vi "Lin_SCUBoot.vi"() -> (2 "Data":T1 {"payload" format="%02x"; "identifier" format="%x"})   [LabVIEW 2018]
uses:
  Crl/LIN_DataType.ctl
panel:
  # "ms"
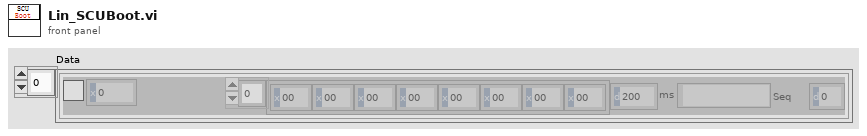
[diagram p1: front panel]
types:
  T1 = typedef "LIN_DataType.ctl" = cluster{"identifier":u32, "payload":u8[], "Send?":bool, "Note":string, "Delays":u32, "Seq":i32}[]
  T2 = cluster{"identifier":u32, "payload":u8[], "Send?":bool, "Note":string, "Delays":u32, "Seq":i32}
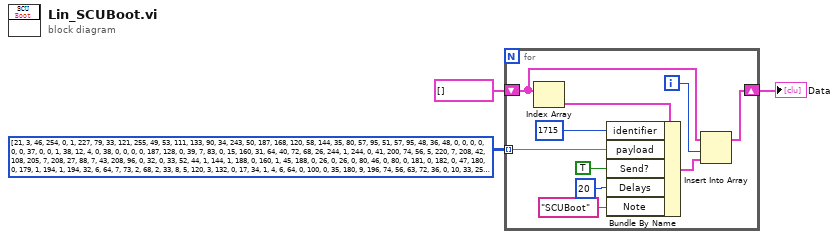
[diagram p0: block diagram]
diagram:
  n1 = for {
    tunnel: u8[][] [[21, 3, 46, 254, 0, 1, 227, 79], [33, 121, 255, 49, 53, 111, 133, 90], [34, 243, 50, 187, 168, 120, 58, 144], [35, 80, 57, 95, 51, 57, 95, 48], [36, 48, 0, 0, 0, 0, 0, 0], [37, 0, 0, 1, 38, 12, 4, 0], [38, 0, 0, 0, 0, 187, 128, 0], [39, 7, 83, 0, 15, 160, 31, 64], [40, 72, 68, 26, 244, 1, 244, 0], [41, 200, 74, 56, 5, 220, 7, 208], [42, 108, 205, 7, 208, 27, 88, 7], [43, 208, 96, 0, 32, 0, 33, 52], [44, 1, 144, 1, 188, 0, 160, 1], [45, 188, 0, 26, 0, 26, 0, 80], [46, 0, 80, 0, 181, 0, 182, 0], [47, 180, 0, 179, 1, 194, 1, 194], [32, 6, 64, 7, 73, 2, 68, 2], [33, 8, 5, 120, 3, 132, 0, 17], [34, 1, 4, 6, 64, 0, 100, 0], [35, 180, 9, 196, 74, 56, 63, 72], [36, 0, 10, 33, 252, 1, 244, 4], [37, 26, 70, 80, 63, 72, 34, 196], [38, 6, 64, 26, 244, 58, 152, 0], [39, 10, 39, 16, 0, 250, 255, 10], [40, 32, 2, 1, 0, 10, 2, 1], [41, 3, 1, 1, 1, 2, 2, 3], [42, 40, 8, 8, 165, 19, 130, 140], [43, 15, 126, 3, 3, 9, 9, 160], [44, 0, 100, 0, 40, 255, 216, 0], [45, 17, 6, 152, 93, 192, 6, 12], [46, 192, 0, 0, 100, 0, 15, 255], [47, 216, 0, 17, 8, 245, 93, 192], [32, 6, 12, 224, 0, 19, 136, 0], [33, 40, 255, 216, 0, 15, 18, 237], [34, 125, 0, 6, 12, 224, 0, 1], [35, 144, 117, 139, 142, 225, 10, 14], [36, 109, 6, 222, 88, 74, 170, 110], [37, 202, 234, 0, 1, 74, 0, 250], [38, 50, 50, 23, 112, 70, 80, 0], [39, 90, 0, 255, 5, 0, 0, 0], [40, 0, 0, 0, 150, 1, 144, 50], [41, 50, 0, 0, 0, 0, 0, 0], [42, 0, 255, 30, 0, 0, 0, 0], [43, 0, 1, 74, 0, 250, 50, 50], [44, 0, 0, 0, 0, 0, 130, 0], [45, 255, 30, 0, 0, 0, 0, 0], [46, 0, 75, 0, 0, 55, 255, 0], [47, 0, 0, 0, 0, 0, 0, 255], [32, 10, 0, 0, 0, 0, 0, 6], [33, 152, 0, 180, 50, 50, 0, 0], [34, 0, 0, 0, 130, 0, 255, 5], [35, 0, 0, 0, 0, 0, 0, 180], [36, 0, 45, 50, 50, 0, 0, 0], [37, 0, 0, 90, 0, 255, 10, 0], [38, 0, 0, 0, 0, 0, 180, 0], [39, 45, 50, 50, 0, 0, 0, 0], [40, 0, 110, 0, 255, 30, 0, 0], [41, 0, 0, 0, 0, 100, 0, 55], [42, 0, 55, 0, 0, 0, 0, 0], [43, 0, 0, 255, 250, 3, 0, 0], [44, 0, 0, 0, 180, 0, 45, 50], [45, 50, 0, 0, 0, 0, 0, 105], [46, 0, 255, 10, 0, 0, 0, 0], [47, 0, 0, 180, 0, 45, 50, 50], [32, 0, 0, 0, 0, 0, 140, 0], [33, 255, 10, 0, 0, 0, 0, 0], [34, 6, 152, 0, 180, 50, 50, 0], [35, 0, 0, 0, 0, 140, 0, 255], [36, 10, 0, 0, 0, 0, 0, 0], [37, 185, 0, 100, 0, 50, 0, 0], [38, 0, 0, 0, 0, 0, 255, 10], [39, 0, 40, 0, 0, 0, 0, 245], [40, 0, 140, 0, 55, 0, 0, 0], [41, 0, 0, 0, 0, 255, 15, 120], [42, 50, 0, 0, 0, 0, 180, 3], [43, 132, 50, 50, 23, 112, 0, 0], [44, 0, 140, 0, 255, 40, 0, 0], [45, 0, 0, 0, 0, 55, 0, 40], [46, 0, 55, 0, 0, 0, 0, 0], [47, 0, 0, 255, 5, 0, 0, 0], [32, 0, 0, 6, 134, 0, 120, 0], [33, 45, 0, 0, 0, 0, 0, 0], [34, 0, 255, 8, 2, 2, 0, 0], [35, 0, 75, 100, 60, 0, 0, 42], [36, 4, 220, 0, 157, 0, 145, 0], [37, 20, 0, 0, 0, 0, 3, 32], [38, 31, 64, 9, 196, 33, 192, 0], [39, 70, 0, 0, 0, 70, 0, 0], [40, 0, 70, 0, 0, 0, 70, 0], [41, 0, 0, 200, 6, 64, 0, 45], [42, 0, 150, 117, 48, 0, 100, 0], [43, 0, 0, 0, 16, 0, 0, 70], [44, 0, 0, 0, 70, 0, 0, 0], [45, 70, 0, 0, 0, 70, 0, 0], [46, 58, 152, 39, 16, 255, 190, 1], [47, 72, 11, 184, 6, 134, 1, 44], [32, 0, 185, 0, 60, 0, 0, 50], [33, 200, 0, 0, 6, 64, 0, 0], [34, 0, 100, 0, 0, 0, 120, 0], [35, 120, 0, 200, 0, 0, 0, 180], [36, 15, 0, 0, 180, 0, 0, 25], [37, 0, 1, 104, 0, 180, 35, 0], [38, 128, 0, 62, 128, 12, 205, 0], [39, 0, 243, 51, 0, 100, 0, 55], [40, 0, 0, 1, 7, 1, 7, 1], [41, 7, 0, 100, 0, 100, 2, 0], [42, 0, 128, 14, 16, 15, 160, 12], [43, 128, 62, 128, 0, 1, 4, 1], [44, 1, 4, 2, 3, 3, 2, 4], [45, 4, 4, 2, 4, 7, 20, 25], [46, 20, 5, 255, 2, 5, 20, 0], [47, 34, 253, 40, 30, 50, 30, 20], [32, 0, 40, 5, 15, 20, 12, 0], [33, 15, 100, 15, 80, 95, 2, 25], [34, 58, 14, 8, 10, 6, 6, 0], [35, 6, 140, 40, 25, 10, 25, 25], [36, 35, 45, 1, 34, 255, 255, 2], [37, 145, 145, 2, 4, 2, 200, 0], [38, 10, 24, 25, 50, 9, 50, 9], [39, 14, 10, 4, 50, 0, 8, 16], [40, 10, 10, 0, 0, 4, 2, 5], [41, 5, 1, 1, 0, 1, 2, 1], [42, 5, 1, 4, 100, 255, 255, 140], [43, 255, 20, 0, 1, 1, 15, 0], [44, 1, 220, 140, 0, 25, 2, 135], [45, 37, 1, 15, 15, 2, 139, 55], [46, 0, 0, 0, 0, 0, 0, 0], [47, 0, 0, 20, 0, 0, 0, 0], [32, 3, 32, 31, 64, 0, 0, 37], [33, 128, 0, 70, 0, 0, 0, 70], [34, 0, 0, 0, 70, 0, 0, 0], [35, 70, 0, 0, 0, 20, 7, 208], [36, 0, 0, 0, 0, 117, 48, 0], [37, 100, 0, 0, 0, 0, 16, 0], [38, 0, 70, 0, 0, 0, 70, 0], [39, 0, 0, 70, 0, 0, 0, 70], [40, 0, 0, 58, 152, 39, 16, 255], [41, 190, 1, 72, 11, 184, 8, 202], [42, 0, 100, 0, 0, 0, 0, 0], [43, 0, 50, 200, 3, 32, 1, 64], [44, 0, 0, 0, 100, 0, 0, 0], [45, 120, 0, 120, 0, 200, 0, 0], [46, 0, 0, 255, 0, 0, 0, 0], [47, 0, 255, 0, 0, 0, 0, 0], [32, 255, 0, 128, 0, 62, 228, 12], [33, 205, 23, 112, 243, 51, 0, 100], [34, 0, 100, 19, 136, 0, 125, 0], [35, 125, 0, 50, 0, 125, 0, 100], [36, 2, 0, 0, 128, 14, 16, 15], [37, 160, 12, 128, 62, 128, 0, 1], [38, 4, 1, 1, 4, 2, 3, 3], [39, 2, 8, 8, 4, 1, 4, 7], [40, 20, 0, 0, 20, 255, 2, 0], [41, 20, 0, 34, 253, 10, 2, 50], [42, 20, 20, 0, 0, 2, 0, 0], [43, 12, 0, 13, 10, 0, 0, 95], [44, 5, 25, 0, 20, 8, 15, 0], [45, 0, 0, 2, 140, 40, 30, 30], [46, 0, 0, 25, 10, 1, 55, 255], [47, 255, 2, 0, 0, 255, 255, 2], [32, 200, 0, 10, 20, 15, 100, 19], [33, 100, 19, 14, 10, 4, 36, 0], [34, 8, 16, 10, 10, 0, 0, 4], [35, 2, 5, 5, 1, 1, 0, 1], [36, 2, 1, 5, 1, 4, 100, 255], [37, 30, 255, 255, 20, 0, 1, 5], [38, 5, 0, 1, 220, 140, 0, 25], [39, 2, 135, 37, 1, 15, 15, 2], [40, 136, 55, 0, 0, 0, 0, 0], [41, 0, 0, 0, 0, 0, 0, 0], [42, 0, 0, 0, 0, 0, 0, 0], [43, 0, 0, 0, 0, 0, 0, 0], [44, 0, 0, 0, 0, 0, 0, 0], [45, 0, 0, 0, 0, 0, 0, 0], [46, 0, 0, 0, 0, 0, 0, 0], [47, 0, 0, 0, 0, 0, 0, 0], [32, 0, 0, 0, 0, 0, 0, 0], [33, 0, 0, 0, 0, 0, 0, 0], [34, 0, 0, 0, 0, 0, 0, 0], [35, 0, 0, 0, 0, 0, 0, 0], [36, 0, 0, 0, 0, 0, 0, 0], [37, 0, 0, 0, 0, 0, 0, 0], [38, 0, 0, 0, 0, 0, 0, 0], [39, 0, 0, 0, 0, 0, 0, 0]] ("目标报文") -> [w12] mode=indexing
    shift-right: [w8] -> w2
    shift-left: T1 [] ("Data") -> [w7]
    i -> [w10]
    n2 = Index Array(array=w7) -> (element=w6:T2)  [unwired: 1 in]
    n3 = Bundle By Name(cluster=w6, "identifier"=u32 1715, "payload"=w12, "Send?"=TRUE, "Delays"=u32 20, "Note"="SCUBoot") -> (w9:T2)
    n4 = Insert Into Array(array=w7, index=w10, new element=w9) -> (w8:T1)
  }
  "Data" <- w2
